vi "BMP zapis parametry.vi"(8 "error in (no error)":errorcluster, 11 "Katalog":path) -> (0 "error out":errorcluster, 1 "OK?":bool, 2 "linie out":bool, 3 "Katalog out":path)   [LabVIEW 2014]
doc: "wybiera lokalizacjê i nazwê pliku BMP"
panel:
  in  "Rysuj linie siatki":bool=TRUE
  in  "Cancel":bool
  in  "OK":bool
  in  "Nazwa pliku BMP":string
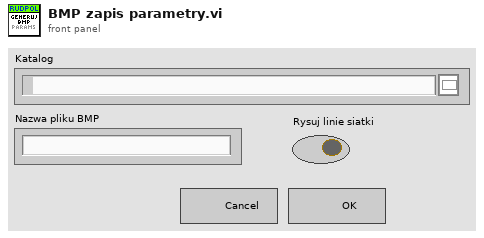
[diagram p1: front panel]
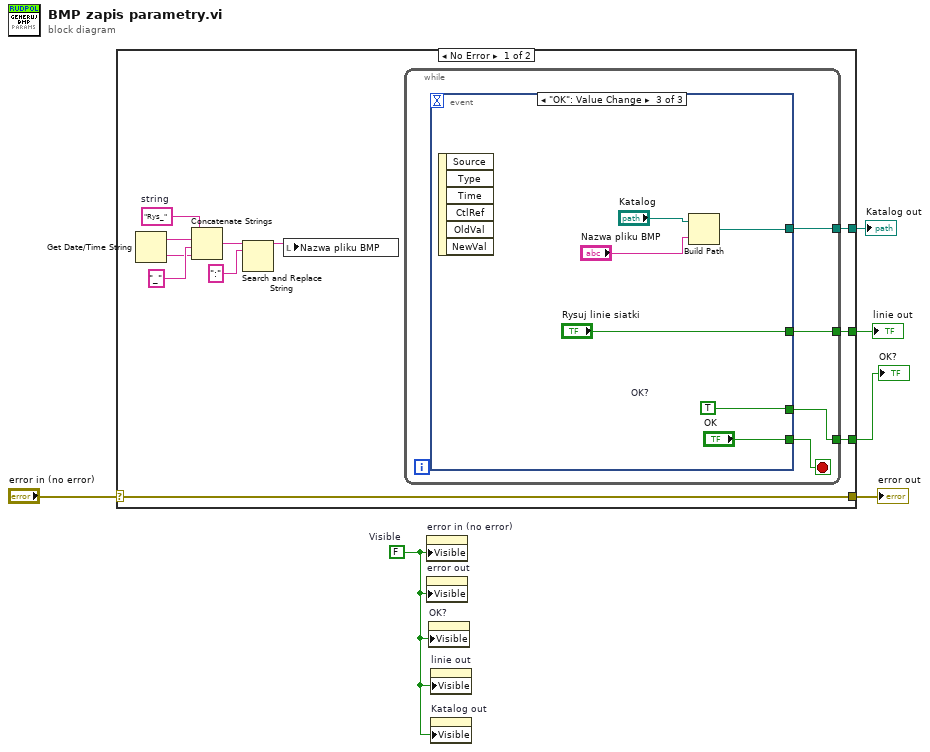
[diagram p0: block diagram]
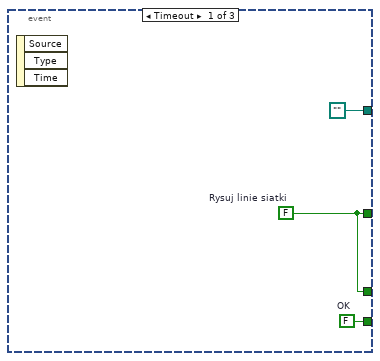
[diagram p2: hidden frame]
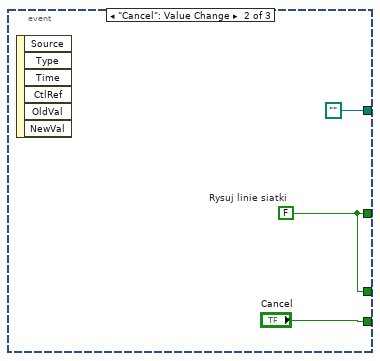
[diagram p3: hidden frame]
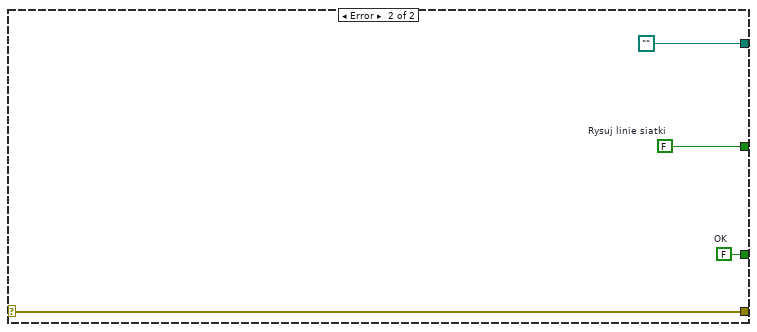
[diagram p4: hidden frame]
diagram:
  w1 = FALSE  # Visible
  n1 = case shown="No Error" "error in (no error)" {
    selector: "error in (no error)" -> [w17 w37]
    tunnel: [w17 w37] -> w5
    tunnel: [w16 w36] -> w4
    tunnel: [w15 path ""] -> w3
    tunnel: [w14 w34] -> w2
    frame No Error {
      w8 = "Rys_"  # string
      n2 = Get Date/Time String() -> (date string=w7:string, time string=w9:string)  [unwired: 3 in]
      n3 = Concatenate Strings(w8, w7, "_" ("string"), w9) -> (w11:string)
      n4 = Search and Replace String(input string=w11, search string=":") -> (result string=w13:string)  [unwired: 6 in, 3 out]
      n5 = local write "Nazwa pliku BMP"(w13) -> ()
      n6 = while {
        tunnel: [w18] -> w16
        tunnel: [w20] -> w15
        tunnel: [w19] -> w14
        stop <- w21 stop-if-true
        n7 = event shown="[2] \"OK\": Value Change" {
          selector: _ -> [_ _ _]
          dyn-events: _ -> [_ _ _]
          timeout: _ -> [_ _ _]
          tunnel: [w24 "Cancel" "OK"] -> w21
          tunnel: [path "" path "" w30] -> w20
          tunnel: [w22 w25 "Rysuj linie siatki"] -> w19
          tunnel: [w22 w25 w29] -> w18
          event Timeout {
            w22 = FALSE  # Rysuj linie siatki
            w24 = FALSE  # OK
            n8 = event-data() -> ()  [unwired: 1 in, 3 out]
          }
          event "Cancel": Value Change {
            w25 = FALSE  # Rysuj linie siatki
            n9 = event-data() -> ()  [unwired: 1 in, 6 out]
          }
          event "OK": Value Change {
            w29 = TRUE  # OK?
            n10 = event-data() -> ()  [unwired: 1 in, 6 out]
            n11 = Build Path(base path="Katalog", name or relative path="Nazwa pliku BMP") -> (appended path=w30:path)
          }
        }
      }
    }
    frame Error {
      w34 = FALSE  # Rysuj linie siatki
      w36 = FALSE  # OK
    }
  }
  "error out" <- w5
  "OK?" <- w4
  "Katalog out" <- w3
  "linie out" <- w2
  n12 = property on="error in (no error)" class="Clust (strict)"("Visible"=w1) -> ()  [unwired: 2 in, 2 out]
  n13 = property on="error out" class="Clust (strict)"("Visible"=w1) -> ()  [unwired: 2 in, 2 out]
  n14 = property on="OK?" class="Bool (strict)"("Visible"=w1) -> ()  [unwired: 2 in, 2 out]
  n15 = property on="linie out" class="Bool (strict)"("Visible"=w1) -> ()  [unwired: 2 in, 2 out]
  n16 = property on="Katalog out" class="Path"("Visible"=w1) -> ()  [unwired: 2 in, 2 out]
